vi "SVPO Convert to Even Angle Signal (1 Ch DBL WDT).vi"(0 "scaled signal [EU]":waveform(dbl)={"t0"=timestamp(0 s since 1904-01-01), "dt"=0.0, "Y"=[]}, 2 "reset? (F)":bool, 7 "speed position info":T1, 12 "max order":dbl=16.0) -> (4 "even-angle signal":cluster{"r0":dbl, "dr":dbl, "Y":dbl[]}={"r0"=0.0, "dr"=1.0, "Y"=[]} {"r0" format="%.2p"; "dr" format="%.2p"; "Y" format="%.2f"}, 8 "even-angle position info":T1)   [LabVIEW 2017, in "SoundVib_OrderTracking.lvlib"]
doc: "Converts an even-time-spaced scaled signal to an even-angle-spaced signal by resampling the acquired signal. The output signal is synchronous to the rotational speed with a constant number of samples per revolution. Use this VI on embedded targets that have limited computational resources. Wire data to the <B>scaled signal [EU]</B> input to determine the polymorphic instance to use or manually select the instance."
uses:
  <vilib>/addons/Sound and Vibration/Order Analysis/Resample Order Tracking/SoundVib_OrderTracking.lvlib
  <vilib>/addons/Sound and Vibration/Order Analysis/Misc/OAT Position Info.ctl
  <vilib>/addons/Sound and Vibration/Order Analysis/Resample Order Tracking/SVPO Convert to Even Angle Signal (1 Ch DBL Array) with IC.vi
  <vilib>/addons/Sound and Vibration/Order Analysis/Resample Order Tracking/SubVIs/sv_Convert to Even Angle Signal (Generic) with IC.vi
  <vilib>/addons/Sound and Vibration/Order Analysis/Adv Resampling/oa_CIC Interpolation Filter with IC.vi
  <vilib>/addons/Sound and Vibration/Order Analysis/Adv Resampling/sv_Resample (Const to Variable, DBL Array) with IC.vi
  <vilib>/addons/Sound and Vibration/Order Analysis/Adv Resampling/sv_Resample Filter Prototype Design.vi
  <vilib>/addons/Sound and Vibration/Order Analysis/Adv Resampling/oa_Adjust Resample State Info.vi
  <vilib>/addons/Sound and Vibration/Order Analysis/Adv Resampling/OAT LP Kaiser Window Design.vi
  <vilib>/addons/Sound and Vibration/Order Analysis/Resample Order Tracking/SubVIs/oa_CIC Filter Length.vi
  <vilib>/addons/Sound and Vibration/Order Analysis/Adv Resampling/sv_Get Actual Max Order.vi
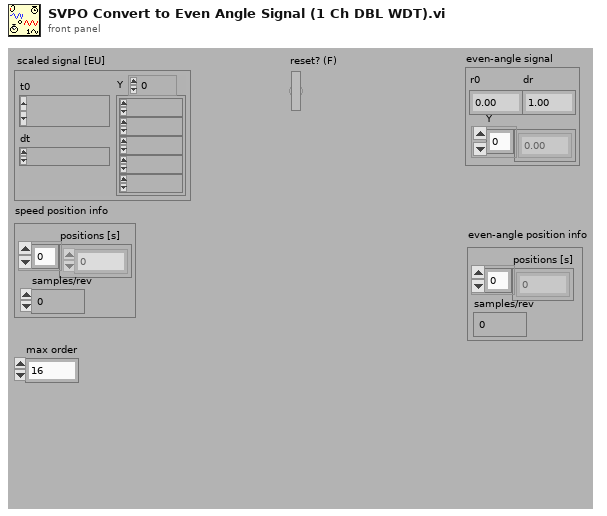
[diagram p1: front panel]
types:
  T1 = typedef "OAT Position Info.ctl" = cluster{"positions [s]":dbl[], "samples/rev":dbl}
  T2 = typedef "svc_Convert to Even Angle State.ctl" = cluster{"filter prototype":T3, "interpolation filter state":cluster{"corrected lengths":i32[], "initH":cluster{"t":dbl[]}[]}, "resample state":cluster{"signal length":u64, "time":dbl[], "reset state":bool, "state":cluster{"init condition":dbl[], "start index":i32, "channel count":i32, "condition len":i32, "position":dbl, "time interval":dbl, "max cond len":i32}, "offset":dbl}}
  T3 = typedef "OAT Resample Filter Prototype.ctl" = cluster{"left wing":dbl[], "increment":dbl[], "max dec":i32, "timing jitter":enum32{"Interpolation", "Rounding"}, "band limiting?":bool}
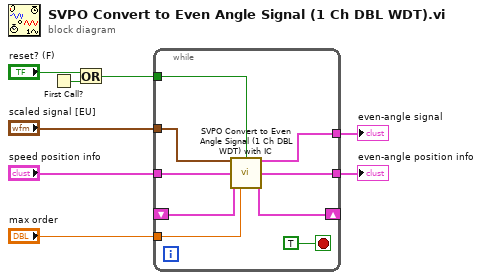
[diagram p0: block diagram]
diagram:
  n1 = First Call?() -> (First Call?: T/F=w7:bool)
  n2 = Or(x="reset? (F)", y=w7) -> (x .or. y?=w6:bool)
  n3 = while {
    tunnel: w6 -> [w17]
    tunnel: "speed position info" -> [w16]
    tunnel: "max order" -> [w15]
    tunnel: [w14] -> w3
    tunnel: [w13] -> w2
    tunnel: "scaled signal [EU]" -> [w12]
    shift-right: [w10] -> _
    shift-left: _ -> [w9]
    stop <- TRUE stop-if-true
    n4 = call <vilib>:"SVPO Convert to Even Angle Signal (1 Ch DBL WDT) with IC.vi"("scaled signal [EU]"=w12, "reset? (F)"=w17, "speed position info"=w16, "initial conditions"=w9, "max order"=w15) -> ("even-angle signal"=w14:cluster{"r0":dbl, "dr":dbl, "Y":dbl[]}, "even-angle position info"=w13:T1, "final conditions"=w10:T2)  [unwired: 8 in]
  }
  "even-angle signal" <- w3
  "even-angle position info" <- w2
